vi "LVLVBoolean.vi"() -> ()   [LabVIEW 2014]
doc: "This function performs an AND of the input values and returns the inverse of the result.\n\nFor information on the data types used for the DLL function, right-click on the Call Library Function node and choose Configure."
uses:
  CLF_Example.dll
panel:
  out "output":bool
  in  "input":bool
  # "See the block diagram for more information."
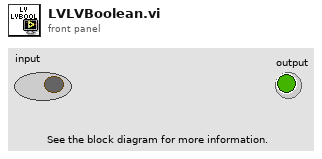
[diagram p1: front panel]
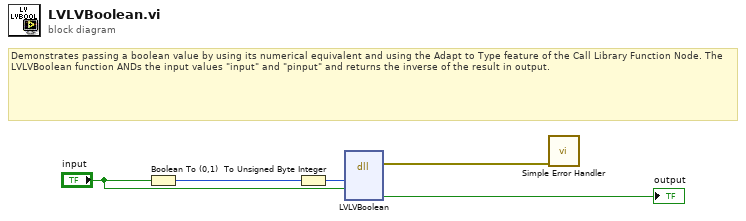
[diagram p0: block diagram]
diagram:
  # "Demonstrates passing a boolean value by using its numerical equivalent and using the Adapt to Type feature of the Call Library Function Node. The LVLVBoolean function ANDs the input values \"input\" and \"pinput\" and returns the inverse of the result in output."
  n1 = Boolean To (0,1)(Boolean="input") -> (0, 1=w4:i16)
  n2 = To Unsigned Byte Integer(number=w4) -> (unsigned 8bit integer=w3:u8)
  n3 = dll-call lib="e:/builds/penguin/labview/branches/2014/dev/dist/examples/Connectivity/Libraries and Executables/DLL Calling VIs/CLF_Example**.*" fn="LVLVBoolean"("input"=w3, "pinput"="input") -> (error out=w1:errorcluster, "output"=→"output":bool)  [unwired: 4 in, 4 out]
  n4 = call <vilib>:"Simple Error Handler.vi"("error in (no error)"=w1) -> ()  [unwired: 4 in, 5 out]
